vi "SingleStationGasMeter.vi"() -> ()   [LabVIEW 2014]
uses:
  <vilib>/DAQmx/read.llb/DAQmx Read (Analog 1D DBL NChan 1Samp).vi
panel:
  out "Meter 6 Present":bool
  out "Meter 5 Present":bool
  out "Meter 4 Present":bool
  out "Meter 3 Present":bool
  out "Meter 2 Present":bool
  out "Meter 1 Present":bool
  out "Meter Type 6":string
  out "Meter Type 2":string
  out "Meter Type 4":string
  out "Meter Type 5":string
  out "Meter Type 3":string
  out "Meter Type 1":string
  out "Meter 6 Size":dbl
  out "Meter 5 Size":dbl
  out "Meter 4 Size":dbl
  out "Meter 3 Size":dbl
  out "Meter 2 Size":dbl
  out "Meter 1 Size":dbl
  out "ANSI Placeholder":dbl
  out "Start Time ANSI":dbl
  in  "Start ANSI":bool
  out "ANSI 5 Minute Average (BTU/hr)":dbl format="%#_5g"
  out "30 Second Average (BTU/hr)":dbl format="%#_5g"
  out "15 Second Average (BTU/hr)":dbl format="%#_5g"
  out "Reference6":dbl
  out "Reference5":dbl
  out "Reference4":dbl
  out "Reference3":dbl
  out "Reference2":dbl
  out "Reference1":dbl
  out "Time":dbl
  out "Num Record":dbl
  in  "HeatingValueLP":dbl=2450.0 min=2400.0 max=2600.0 step=5.0
  out "Output 6":dbl min=0.0 max=5.0 step=0.01
  out "Output 5":dbl min=0.0 max=5.0 step=0.01
  out "Output 4":dbl min=0.0 max=5.0 step=0.01
  out "Output 3":dbl min=0.0 max=5.0 step=0.01
  out "Output 2":dbl min=0.0 max=5.0 step=0.01
  out "Output 1":dbl min=0.0 max=5.0 step=0.01
  out "Signal":bool
  in  "Record":bool
  out "File Path":path
  out "CF/HR":dbl format="%#_2g"
  out "HV":dbl
  in  "HeatingValueNG":dbl=990.0 min=990.0 max=1150.0 step=1.0
  out "Meter ID":dbl
  out "Gas":string
  out "DisplayChart":cluster{"Flow Rate":dbl}(graph)
  out "Flow Rate":dbl format="%#_5g"
  # "Instant Flow Rate (BTU/hr)"
  # "Heating Value"
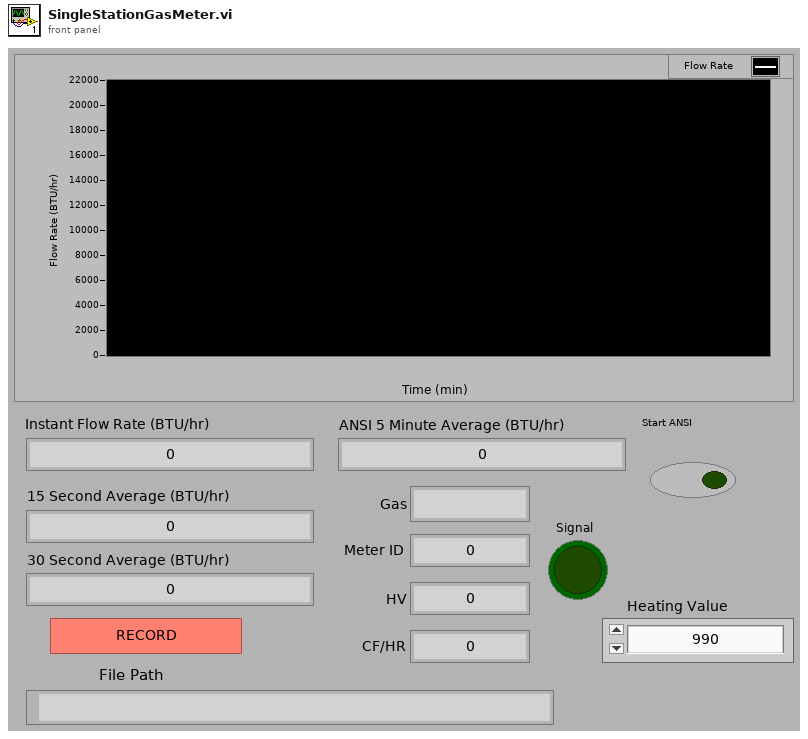
[diagram p1: front panel]
types:
  T1 = enum16{"open", "replace", "create", "open or create", "replace or create", "replace or create with confirmation"}
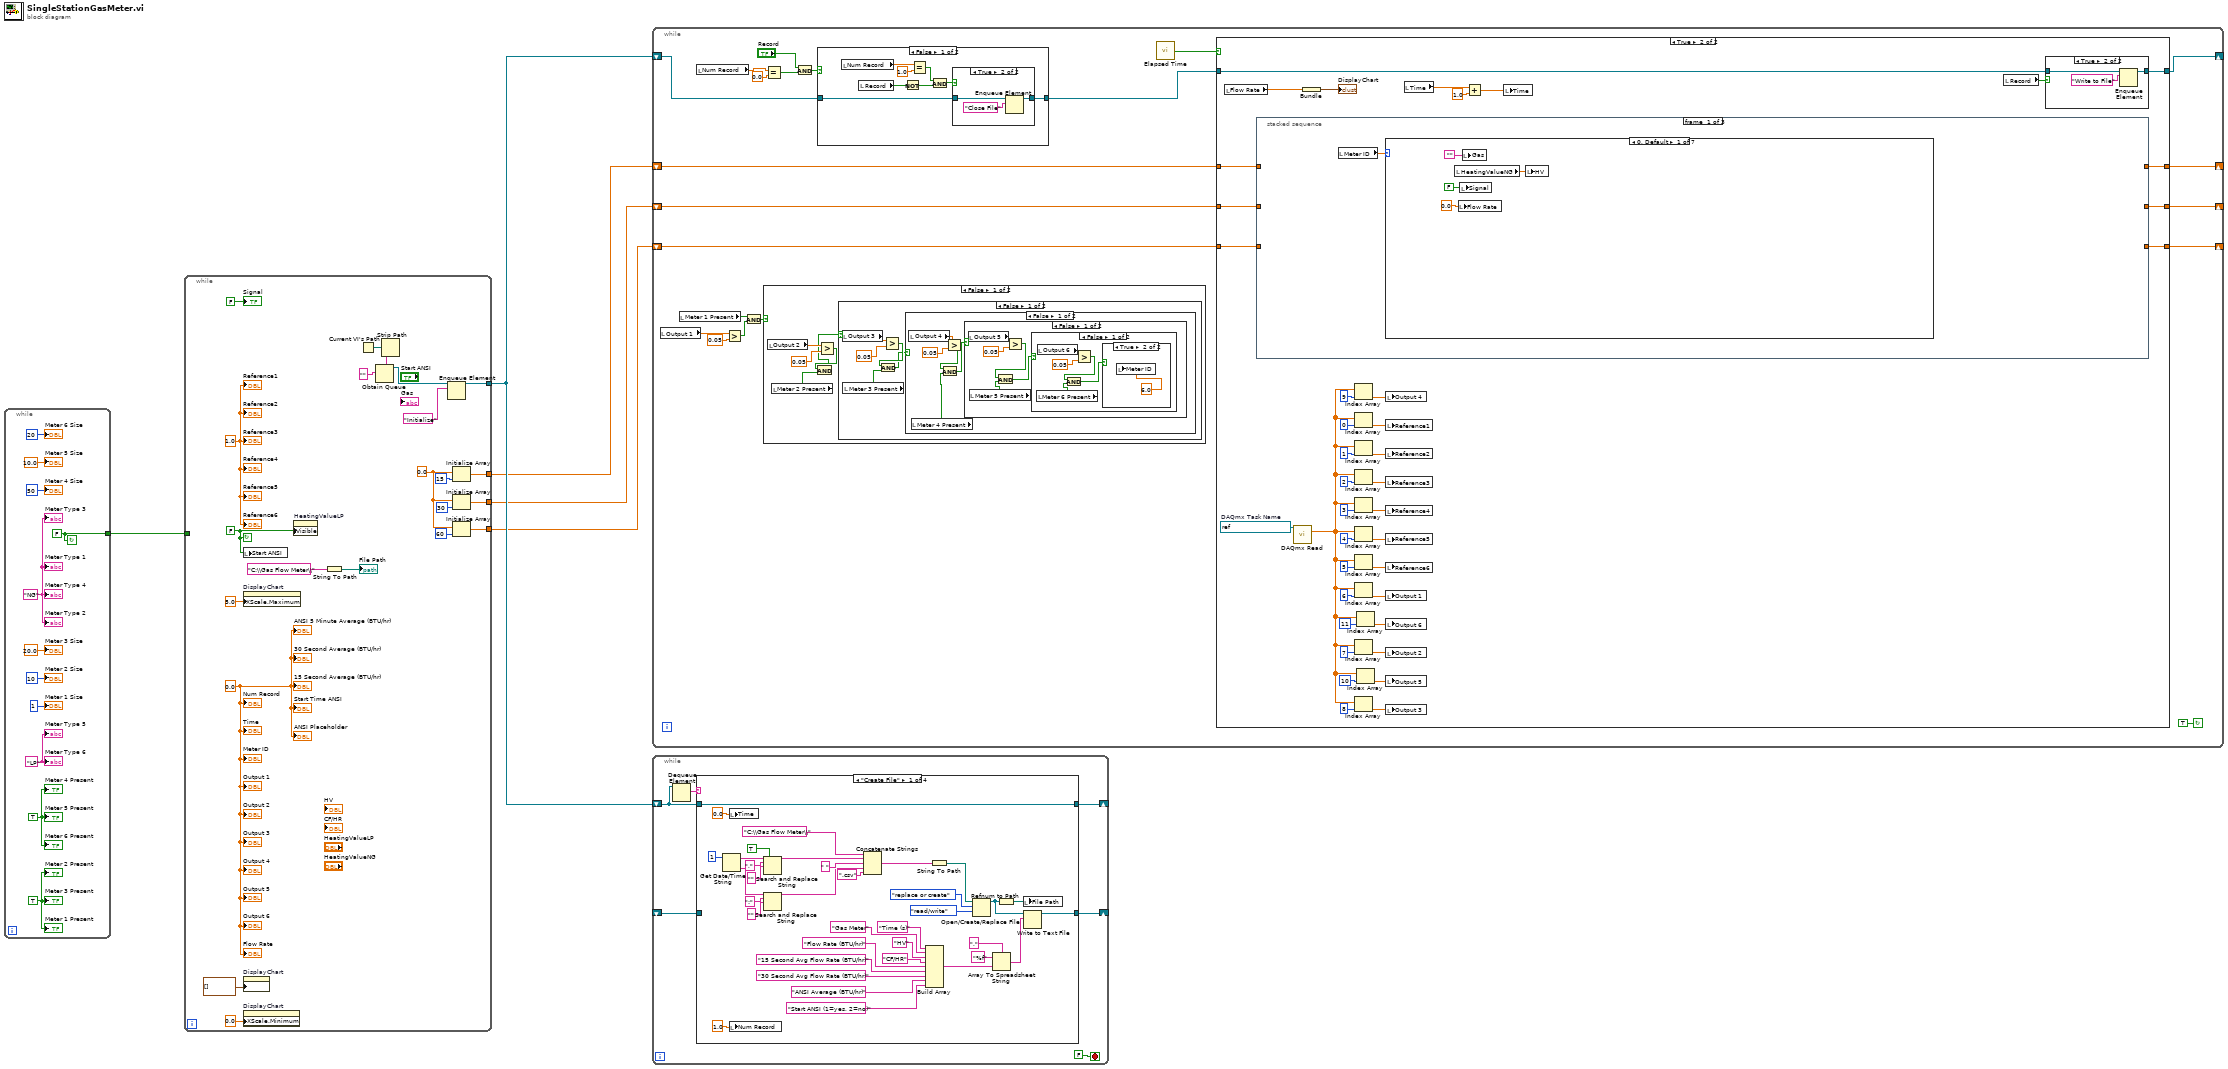
[diagram p0: block diagram]
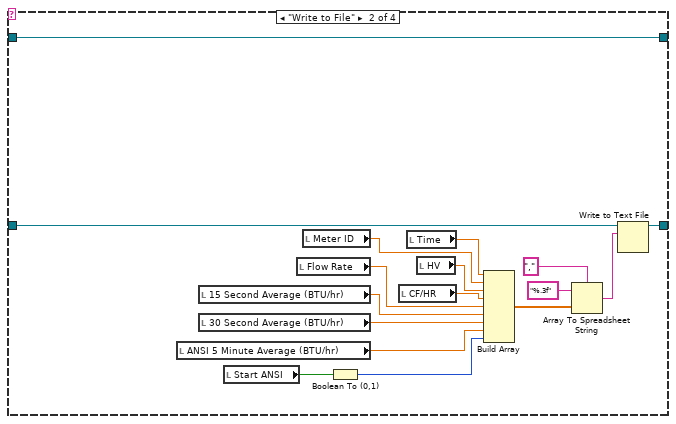
[diagram p2: hidden frame]
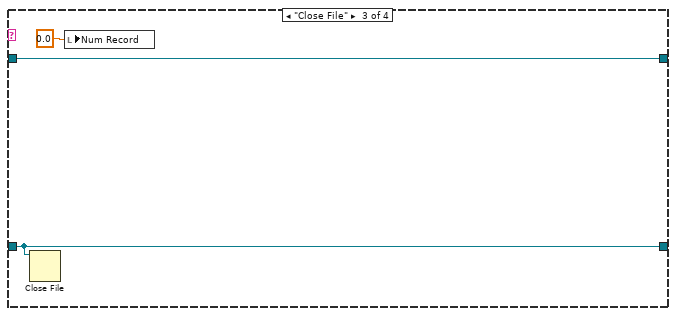
[diagram p3: hidden frame]
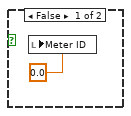
[diagram p5: hidden frame]
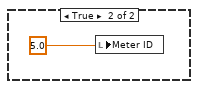
[diagram p6: hidden frame]
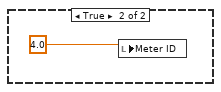
[diagram p7: hidden frame]
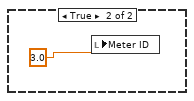
[diagram p8: hidden frame]
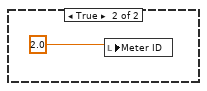
[diagram p9: hidden frame]
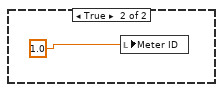
[diagram p10: hidden frame]
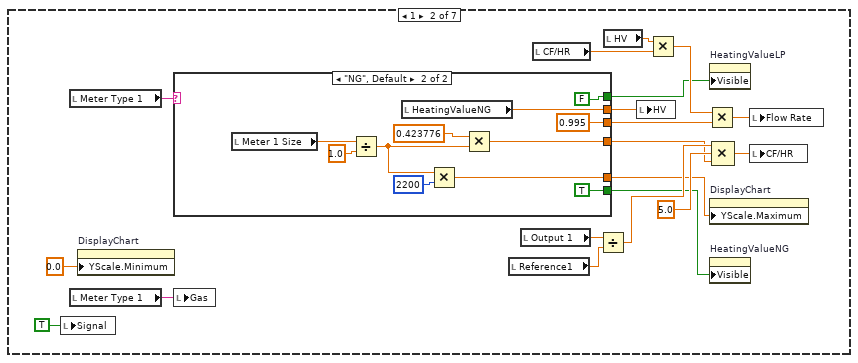
[diagram p12: hidden frame]
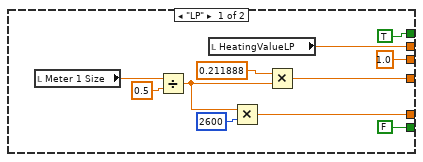
[diagram p13: hidden frame]
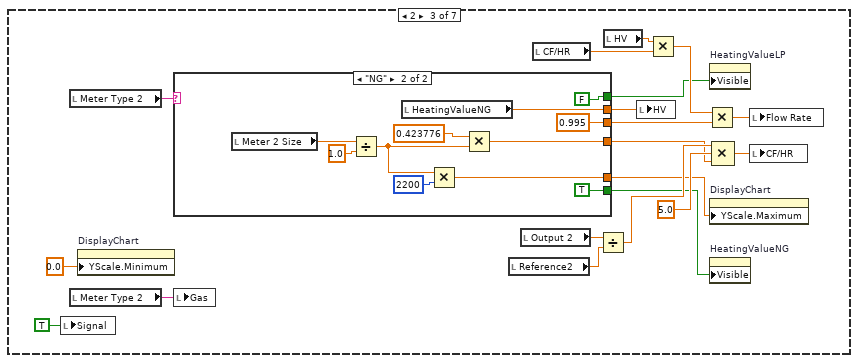
[diagram p14: hidden frame]
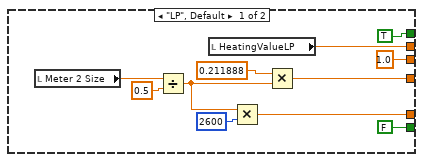
[diagram p15: hidden frame]
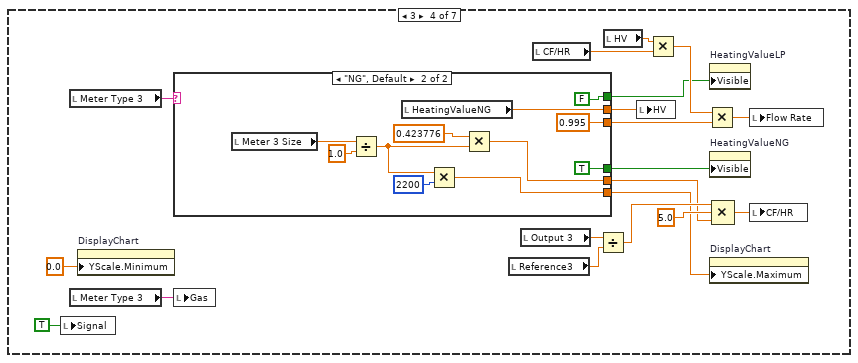
[diagram p16: hidden frame]
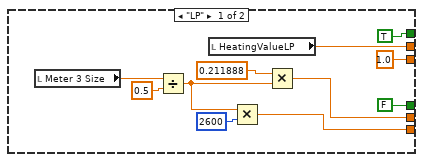
[diagram p17: hidden frame]
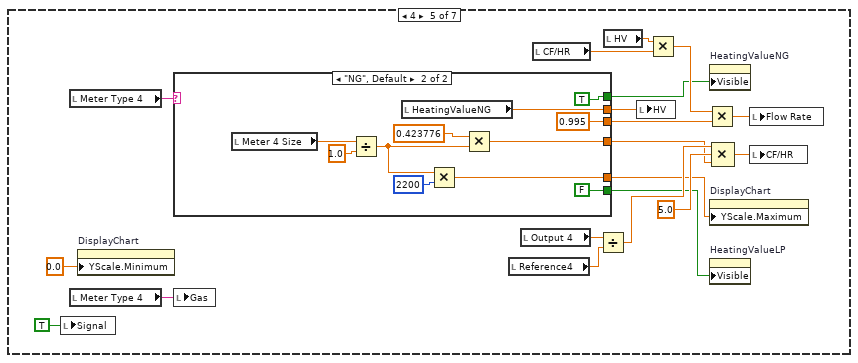
[diagram p18: hidden frame]
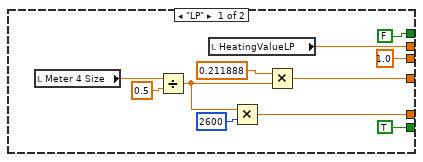
[diagram p19: hidden frame]
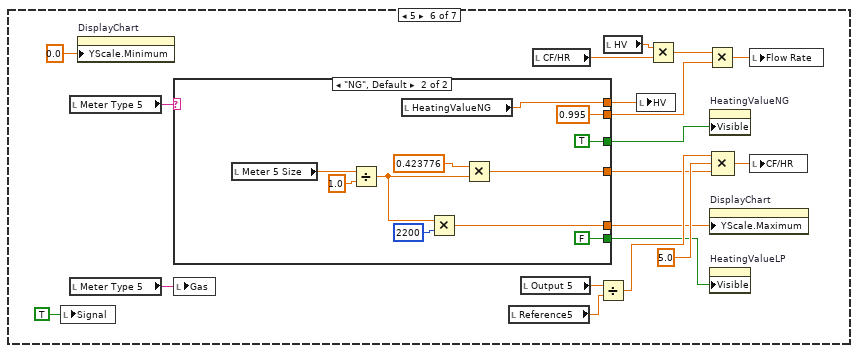
[diagram p20: hidden frame]
diagram:
  n1 = while {
    tunnel: [w16] -> w1
    stop <- w16 continue-if-true
    w13 = "LP"
    w6 = "NG"
    w14 = TRUE
    w15 = TRUE
    w16 = FALSE
    "Meter 4 Size" <- 50
    "Meter 5 Size" <- 10.0
    "Meter 2 Size" <- 10
    "Meter 1 Size" <- 1
    "Meter 6 Size" <- 20
    "Meter 3 Size" <- 20.0
    "Meter Type 1" <- w6
    "Meter Type 6" <- w13
    "Meter Type 3" <- w6
    "Meter Type 2" <- w6
    "Meter Type 5" <- w13
    "Meter Type 4" <- w6
    "Meter 1 Present" <- w15
    "Meter 2 Present" <- w15
    "Meter 3 Present" <- w15
    "Meter 4 Present" <- w14
    "Meter 5 Present" <- w14
    "Meter 6 Present" <- w14
  }
  n2 = while {
    tunnel: [w30] -> w5
    tunnel: [w24] -> w4
    tunnel: [w23] -> w3
    tunnel: [w20] -> w2
    tunnel: w1 -> [_]
    stop <- w19 continue-if-true
    w22 = 0.0
    w29 = 1.0
    w18 = 0.0
    w19 = FALSE
    n3 = local write "Start ANSI"(w19) -> ()
    n4 = property on="DisplayChart" class="WFChart (strict)"("XScale.Maximum"=5.0) -> ()  [unwired: 2 in, 2 out]
    n5 = property on="DisplayChart" class="WFChart (strict)"("History Data"=cluster{"[0]":dbl}[] []) -> ()  [unwired: 2 in, 2 out]
    n6 = property on="DisplayChart" class="WFChart (strict)"("XScale.Minimum"=0.0) -> ()  [unwired: 2 in, 2 out]
    n7 = property on="HeatingValueLP" class="DigNum (strict)"("Visible"=w19) -> ()  [unwired: 2 in, 2 out]
    n8 = String To Path(string="C:\\Gas Flow Meter\\") -> (path=→"File Path":path)
    n9 = Current VI's Path() -> (path=w35:path)
    n10 = Strip Path(path=w35) -> (name=w33:string)  [unwired: 1 out]
    n11 = Obtain Queue(name (unnamed)=w33, element data type="") -> (queue out=w31:refnum<queue>)  [unwired: 3 in, 2 out]
    n12 = Enqueue Element(queue=w31, element="Initialize") -> (queue out=w30:refnum<queue>)  [unwired: 2 in, 2 out]
    n13 = Initialize Array(w22, 15) -> (w24:dbl[])
    n14 = Initialize Array(w22, 30) -> (w23:dbl[])
    n15 = Initialize Array(w22, 60) -> (w20:dbl[])
    "Num Record" <- w18
    "Time" <- w18
    "Meter ID" <- w18
    "Output 1" <- w18
    "Output 2" <- w18
    "Output 3" <- w18
    "Output 4" <- w18
    "Output 5" <- w18
    "Output 6" <- w18
    "Reference1" <- w29
    "Reference2" <- w29
    "Reference3" <- w29
    "Reference4" <- w29
    "Reference5" <- w29
    "Reference6" <- w29
    "30 Second Average (BTU/hr)" <- w18
    "15 Second Average (BTU/hr)" <- w18
    "ANSI 5 Minute Average (BTU/hr)" <- w18
    "Start Time ANSI" <- w18
    "ANSI Placeholder" <- w18
    "Flow Rate" <- w18
    "Signal" <- FALSE
  }
  n16 = while {
    shift-right: [w51] -> _
    shift-left: w5 -> [w50]
    shift-right: [w47] -> _
    shift-left: w4 -> [w45]
    shift-right: [w46] -> _
    shift-left: w3 -> [w44]
    shift-right: [w43] -> _
    shift-left: w2 -> [w42]
    stop <- TRUE continue-if-true
    n17 = local read "Output 1"() -> (w49:dbl)
    n18 = local read "Meter 1 Present"() -> (w40:bool)
    n19 = local read "Num Record"() -> (w55:dbl)
    n20 = Greater?(x=w49, y=0.05) -> (0:w41:bool)
    n21 = And(x=w40, y=w41) -> (x .and. y?=w39:bool)
    n22 = case shown="False" w39 {
      frame False {
        n23 = local read "Output 2"() -> (w63:dbl)
        n24 = local read "Meter 2 Present"() -> (w62:bool)
        n25 = Greater?(x=w63, y=0.05) -> (0:w61:bool)
        n26 = And(x=w61, y=w62) -> (x .and. y?=w60:bool)
        n27 = case shown="False" w60 {
          frame False {
            n28 = local read "Output 3"() -> (w68:dbl)
            n29 = local read "Meter 3 Present"() -> (w67:bool)
            n30 = Greater?(x=w68, y=0.05) -> (0:w66:bool)
            n31 = And(x=w66, y=w67) -> (x .and. y?=w65:bool)
            n32 = case shown="False" w65 {
              frame False {
                n33 = local read "Output 4"() -> (w73:dbl)
                n34 = local read "Meter 4 Present"() -> (w72:bool)
                n35 = Greater?(x=w73, y=0.05) -> (0:w71:bool)
                n36 = And(x=w71, y=w72) -> (x .and. y?=w70:bool)
                n37 = case shown="False" w70 {
                  frame False {
                    n38 = local read "Output 5"() -> (w78:dbl)
                    n39 = local read "Meter 5 Present"() -> (w77:bool)
                    n40 = Greater?(x=w78, y=0.05) -> (0:w76:bool)
                    n41 = And(x=w76, y=w77) -> (x .and. y?=w75:bool)
                    n42 = case shown="False" w75 {
                      frame False {
                        n43 = local read "Meter 6 Present"() -> (w82:bool)
                        n44 = local read "Output 6"() -> (w83:dbl)
                        n45 = Greater?(x=w83, y=0.05) -> (0:w81:bool)
                        n46 = And(x=w81, y=w82) -> (x .and. y?=w80:bool)
                        n47 = case shown="True" w80 {
                          frame False {
                            n48 = local write "Meter ID"(0.0) -> ()
                          }
                          frame True {
                            n49 = local write "Meter ID"(6.0) -> ()
                          }
                        }
                      }
                      frame True {
                        n50 = local write "Meter ID"(5.0) -> ()
                      }
                    }
                  }
                  frame True {
                    n51 = local write "Meter ID"(4.0) -> ()
                  }
                }
              }
              frame True {
                n52 = local write "Meter ID"(3.0) -> ()
              }
            }
          }
          frame True {
            n53 = local write "Meter ID"(2.0) -> ()
          }
        }
      }
      frame True {
        n54 = local write "Meter ID"(1.0) -> ()
      }
    }
    n55 = Equal?(x=w55, y=0.0) -> (x = y?=w54:bool)
    n56 = And(x="Record", y=w54) -> (x .and. y?=w53:bool)
    n57 = case shown="False" w53 {
      tunnel: w50 -> [w435 w443]
      tunnel: [w434 w442] -> w52
      frame False {
        n58 = local read "Num Record"() -> (w437:dbl)
        n59 = local read "Record"() -> (w431:bool)
        n60 = Not(x=w431) -> (.not. x?=w430:bool)
        n61 = Equal?(x=w437, y=1.0) -> (x = y?=w433:bool)
        n62 = And(x=w433, y=w430) -> (x .and. y?=w432:bool)
        n63 = case shown="True" w432 {
          tunnel: w435 -> [w438 w440]
          tunnel: [w438 w439] -> w434
          frame False {
          }
          frame True {
            n64 = Enqueue Element(queue=w440, element="Close File") -> (queue out=w439:refnum<queue>)  [unwired: 2 in, 2 out]
          }
        }
      }
      frame True {
        n65 = Enqueue Element(queue=w443, element="Create File") -> (queue out=w442:refnum<queue>)  [unwired: 2 in, 2 out]
      }
    }
    n66 = call "Elapsed Time"() -> ("Time has Elapsed"=w58:bool)  [unwired: 12 in, 7 out]
    n67 = case shown="True" w58 {
      tunnel: w52 -> [w95 w129]
      tunnel: [w95 w128] -> w51
      tunnel: w45 -> [w94 w101]
      tunnel: w44 -> [w93 w100]
      tunnel: [w94 w99] -> w47
      tunnel: [w93 w98] -> w46
      tunnel: w42 -> [w92 w97]
      tunnel: [w92 w96] -> w43
      frame False {
      }
      frame True {
        w127 = refnum<k21> "ReadFlowMeterIn"  # DAQmx Task Name
        n68 = local read "Flow Rate"() -> (w135:dbl)
        n69 = stacked-sequence {
          tunnel: w101 -> [_ w411 _]
          tunnel: w100 -> [_ w410 _]
          tunnel: [_ w405 _] -> w99
          tunnel: [_ w401 _] -> w98
          tunnel: w97 -> [_ w395 _]
          tunnel: [_ w392 _] -> w96
          frame #0 {
            n70 = local read "Meter ID"() -> (w136:dbl)
            n71 = case shown="0, Default" w136 {
              frame 0, Default {
                n72 = local read "HeatingValueNG"() -> (w140:dbl)
                n73 = local write "Flow Rate"(0.0) -> ()
                n74 = local write "Signal"(FALSE) -> ()
                n75 = local write "Gas"("") -> ()
                n76 = local write "HV"(w140) -> ()
              }
              frame 1 {
                n77 = local write "Signal"(TRUE) -> ()
                n78 = local read "Meter Type 1"() -> (w149:string)
                n79 = local read "Meter Type 1"() -> (w143:string)
                n80 = property on="DisplayChart" class="WFChart (strict)"("YScale.Minimum"=0.0) -> ()  [unwired: 2 in, 2 out]
                n81 = case shown="\"NG\", Default" w149 {
                  tunnel: [w167 w178] -> w148
                  tunnel: [TRUE FALSE] -> w147
                  tunnel: [FALSE TRUE] -> w146
                  tunnel: [1.0 0.995] -> w145
                  tunnel: [w161 w172] -> w144
                  tunnel: [w160 w171] -> w142
                  frame "LP" {
                    n82 = local read "Meter 1 Size"() -> (w169:dbl)
                    n83 = Divide(x=w169, y=0.5) -> (x/y=w162:dbl)
                    n84 = local read "HeatingValueLP"() -> (w160:dbl)
                    n85 = Multiply(x=w162, y=2600) -> (x*y=w161:dbl)
                    n86 = Multiply(x=0.211888, y=w162) -> (x*y=w167:dbl)
                  }
                  frame "NG", Default {
                    n87 = local read "Meter 1 Size"() -> (w180:dbl)
                    n88 = Divide(x=w180, y=1.0) -> (x/y=w173:dbl)
                    n89 = local read "HeatingValueNG"() -> (w171:dbl)
                    n90 = Multiply(x=w173, y=2200) -> (x*y=w172:dbl)
                    n91 = Multiply(x=0.423776, y=w173) -> (x*y=w178:dbl)
                  }
                }
                n92 = local write "Gas"(w143) -> ()
                n93 = local read "Reference1"() -> (w153:dbl)
                n94 = local read "Output 1"() -> (w154:dbl)
                n95 = local read "CF/HR"() -> (w156:dbl)
                n96 = Divide(x=w154, y=w153) -> (x/y=w151:dbl)
                n97 = local read "HV"() -> (w155:dbl)
                n98 = local write "HV"(w142) -> ()
                n99 = Multiply(x=w155, y=w156) -> (x*y=w157:dbl)
                n100 = Multiply(x=w157, y=w145) -> (x*y=w158:dbl)
                n101 = property on="HeatingValueLP" class="DigNum (strict)"("Visible"=w147) -> ()  [unwired: 2 in, 2 out]
                n102 = property on="DisplayChart" class="WFChart (strict)"("YScale.Maximum"=w144) -> ()  [unwired: 2 in, 2 out]
                n103 = property on="HeatingValueNG" class="DigNum (strict)"("Visible"=w146) -> ()  [unwired: 2 in, 2 out]
                n104 = Compound Arithmetic op=MULTIPLY(w151, 5.0, w148) -> (w141:dbl)
                n105 = local write "Flow Rate"(w158) -> ()
                n106 = local write "CF/HR"(w141) -> ()
              }
              frame 2 {
                n107 = local write "Signal"(TRUE) -> ()
                n108 = local read "Meter Type 2"() -> (w190:string)
                n109 = local read "Meter Type 2"() -> (w184:string)
                n110 = property on="DisplayChart" class="WFChart (strict)"("YScale.Minimum"=0.0) -> ()  [unwired: 2 in, 2 out]
                n111 = case shown="\"NG\"" w190 {
                  tunnel: [w208 w219] -> w189
                  tunnel: [TRUE FALSE] -> w188
                  tunnel: [FALSE TRUE] -> w187
                  tunnel: [1.0 0.995] -> w186
                  tunnel: [w202 w213] -> w185
                  tunnel: [w201 w212] -> w183
                  frame "LP", Default {
                    n112 = local read "Meter 2 Size"() -> (w210:dbl)
                    n113 = Divide(x=w210, y=0.5) -> (x/y=w203:dbl)
                    n114 = local read "HeatingValueLP"() -> (w201:dbl)
                    n115 = Multiply(x=w203, y=2600) -> (x*y=w202:dbl)
                    n116 = Multiply(x=0.211888, y=w203) -> (x*y=w208:dbl)
                  }
                  frame "NG" {
                    n117 = local read "Meter 2 Size"() -> (w221:dbl)
                    n118 = Divide(x=w221, y=1.0) -> (x/y=w214:dbl)
                    n119 = local read "HeatingValueNG"() -> (w212:dbl)
                    n120 = Multiply(x=w214, y=2200) -> (x*y=w213:dbl)
                    n121 = Multiply(x=0.423776, y=w214) -> (x*y=w219:dbl)
                  }
                }
                n122 = local write "Gas"(w184) -> ()
                n123 = local read "Reference2"() -> (w194:dbl)
                n124 = local read "Output 2"() -> (w195:dbl)
                n125 = local read "CF/HR"() -> (w197:dbl)
                n126 = Divide(x=w195, y=w194) -> (x/y=w192:dbl)
                n127 = local read "HV"() -> (w196:dbl)
                n128 = local write "HV"(w183) -> ()
                n129 = Multiply(x=w196, y=w197) -> (x*y=w198:dbl)
                n130 = Multiply(x=w198, y=w186) -> (x*y=w199:dbl)
                n131 = property on="HeatingValueLP" class="DigNum (strict)"("Visible"=w188) -> ()  [unwired: 2 in, 2 out]
                n132 = property on="DisplayChart" class="WFChart (strict)"("YScale.Maximum"=w185) -> ()  [unwired: 2 in, 2 out]
                n133 = property on="HeatingValueNG" class="DigNum (strict)"("Visible"=w187) -> ()  [unwired: 2 in, 2 out]
                n134 = Compound Arithmetic op=MULTIPLY(w192, 5.0, w189) -> (w182:dbl)
                n135 = local write "Flow Rate"(w199) -> ()
                n136 = local write "CF/HR"(w182) -> ()
              }
              frame 3 {
                n137 = local write "Signal"(TRUE) -> ()
                n138 = local read "Meter Type 3"() -> (w231:string)
                n139 = local read "Meter Type 3"() -> (w225:string)
                n140 = property on="DisplayChart" class="WFChart (strict)"("YScale.Minimum"=0.0) -> ()  [unwired: 2 in, 2 out]
                n141 = case shown="\"NG\", Default" w231 {
                  tunnel: [w249 w260] -> w230
                  tunnel: [TRUE FALSE] -> w229
                  tunnel: [FALSE TRUE] -> w228
                  tunnel: [1.0 0.995] -> w227
                  tunnel: [w243 w254] -> w226
                  tunnel: [w242 w253] -> w224
                  frame "LP" {
                    n142 = local read "Meter 3 Size"() -> (w251:dbl)
                    n143 = Divide(x=w251, y=0.5) -> (x/y=w244:dbl)
                    n144 = local read "HeatingValueLP"() -> (w242:dbl)
                    n145 = Multiply(x=w244, y=2600) -> (x*y=w243:dbl)
                    n146 = Multiply(x=0.211888, y=w244) -> (x*y=w249:dbl)
                  }
                  frame "NG", Default {
                    n147 = local read "Meter 3 Size"() -> (w262:dbl)
                    n148 = Divide(x=w262, y=1.0) -> (x/y=w255:dbl)
                    n149 = local read "HeatingValueNG"() -> (w253:dbl)
                    n150 = Multiply(x=w255, y=2200) -> (x*y=w254:dbl)
                    n151 = Multiply(x=0.423776, y=w255) -> (x*y=w260:dbl)
                  }
                }
                n152 = local write "Gas"(w225) -> ()
                n153 = local read "Reference3"() -> (w235:dbl)
                n154 = local read "Output 3"() -> (w236:dbl)
                n155 = local read "CF/HR"() -> (w238:dbl)
                n156 = Divide(x=w236, y=w235) -> (x/y=w233:dbl)
                n157 = local read "HV"() -> (w237:dbl)
                n158 = local write "HV"(w224) -> ()
                n159 = Multiply(x=w237, y=w238) -> (x*y=w239:dbl)
                n160 = Multiply(x=w239, y=w227) -> (x*y=w240:dbl)
                n161 = property on="HeatingValueLP" class="DigNum (strict)"("Visible"=w229) -> ()  [unwired: 2 in, 2 out]
                n162 = property on="HeatingValueNG" class="DigNum (strict)"("Visible"=w228) -> ()  [unwired: 2 in, 2 out]
                n163 = property on="DisplayChart" class="WFChart (strict)"("YScale.Maximum"=w226) -> ()  [unwired: 2 in, 2 out]
                n164 = Compound Arithmetic op=MULTIPLY(w233, 5.0, w230) -> (w223:dbl)
                n165 = local write "Flow Rate"(w240) -> ()
                n166 = local write "CF/HR"(w223) -> ()
              }
              frame 4 {
                n167 = local write "Signal"(TRUE) -> ()
                n168 = local read "Meter Type 4"() -> (w272:string)
                n169 = local read "Meter Type 4"() -> (w266:string)
                n170 = property on="DisplayChart" class="WFChart (strict)"("YScale.Minimum"=0.0) -> ()  [unwired: 2 in, 2 out]
                n171 = case shown="\"NG\", Default" w272 {
                  tunnel: [w290 w301] -> w271
                  tunnel: [TRUE FALSE] -> w270
                  tunnel: [FALSE TRUE] -> w269
                  tunnel: [1.0 0.995] -> w268
                  tunnel: [w284 w295] -> w267
                  tunnel: [w283 w294] -> w265
                  frame "LP" {
                    n172 = local read "Meter 4 Size"() -> (w292:dbl)
                    n173 = Divide(x=w292, y=0.5) -> (x/y=w285:dbl)
                    n174 = local read "HeatingValueLP"() -> (w283:dbl)
                    n175 = Multiply(x=w285, y=2600) -> (x*y=w284:dbl)
                    n176 = Multiply(x=0.211888, y=w285) -> (x*y=w290:dbl)
                  }
                  frame "NG", Default {
                    n177 = local read "Meter 4 Size"() -> (w303:dbl)
                    n178 = Divide(x=w303, y=1.0) -> (x/y=w296:dbl)
                    n179 = local read "HeatingValueNG"() -> (w294:dbl)
                    n180 = Multiply(x=w296, y=2200) -> (x*y=w295:dbl)
                    n181 = Multiply(x=0.423776, y=w296) -> (x*y=w301:dbl)
                  }
                }
                n182 = local write "Gas"(w266) -> ()
                n183 = local read "Reference4"() -> (w276:dbl)
                n184 = local read "Output 4"() -> (w277:dbl)
                n185 = local read "CF/HR"() -> (w279:dbl)
                n186 = Divide(x=w277, y=w276) -> (x/y=w274:dbl)
                n187 = local read "HV"() -> (w278:dbl)
                n188 = local write "HV"(w265) -> ()
                n189 = Multiply(x=w278, y=w279) -> (x*y=w280:dbl)
                n190 = Multiply(x=w280, y=w268) -> (x*y=w281:dbl)
                n191 = property on="HeatingValueNG" class="DigNum (strict)"("Visible"=w269) -> ()  [unwired: 2 in, 2 out]
                n192 = property on="DisplayChart" class="WFChart (strict)"("YScale.Maximum"=w267) -> ()  [unwired: 2 in, 2 out]
                n193 = property on="HeatingValueLP" class="DigNum (strict)"("Visible"=w270) -> ()  [unwired: 2 in, 2 out]
                n194 = Compound Arithmetic op=MULTIPLY(w274, 5.0, w271) -> (w264:dbl)
                n195 = local write "Flow Rate"(w281) -> ()
                n196 = local write "CF/HR"(w264) -> ()
              }
              frame 5 {
                n197 = local write "Signal"(TRUE) -> ()
                n198 = local read "Meter Type 5"() -> (w313:string)
                n199 = local read "Meter Type 5"() -> (w307:string)
                n200 = property on="DisplayChart" class="WFChart (strict)"("YScale.Minimum"=0.0) -> ()  [unwired: 2 in, 2 out]
                n201 = case shown="\"NG\", Default" w313 {
                  tunnel: [w331 w342] -> w312
                  tunnel: [TRUE FALSE] -> w311
                  tunnel: [FALSE TRUE] -> w310
                  tunnel: [1.0 0.995] -> w309
                  tunnel: [w325 w336] -> w308
                  tunnel: [w324 w335] -> w306
                  frame "LP" {
                    n202 = local read "Meter 5 Size"() -> (w333:dbl)
                    n203 = Divide(x=w333, y=0.5) -> (x/y=w326:dbl)
                    n204 = local read "HeatingValueLP"() -> (w324:dbl)
                    n205 = Multiply(x=w326, y=2600) -> (x*y=w325:dbl)
                    n206 = Multiply(x=0.211888, y=w326) -> (x*y=w331:dbl)
                  }
                  frame "NG", Default {
                    n207 = local read "Meter 5 Size"() -> (w344:dbl)
                    n208 = Divide(x=w344, y=1.0) -> (x/y=w337:dbl)
                    n209 = local read "HeatingValueNG"() -> (w335:dbl)
                    n210 = Multiply(x=w337, y=2200) -> (x*y=w336:dbl)
                    n211 = Multiply(x=0.423776, y=w337) -> (x*y=w342:dbl)
                  }
                }
                n212 = local write "Gas"(w307) -> ()
                n213 = local read "Reference5"() -> (w317:dbl)
                n214 = local read "Output 5"() -> (w318:dbl)
                n215 = local read "CF/HR"() -> (w320:dbl)
                n216 = Divide(x=w318, y=w317) -> (x/y=w315:dbl)
                n217 = local read "HV"() -> (w319:dbl)
                n218 = local write "HV"(w306) -> ()
                n219 = Multiply(x=w319, y=w320) -> (x*y=w321:dbl)
                n220 = Multiply(x=w321, y=w309) -> (x*y=w322:dbl)
                n221 = property on="HeatingValueNG" class="DigNum (strict)"("Visible"=w310) -> ()  [unwired: 2 in, 2 out]
                n222 = property on="DisplayChart" class="WFChart (strict)"("YScale.Maximum"=w308) -> ()  [unwired: 2 in, 2 out]
                n223 = property on="HeatingValueLP" class="DigNum (strict)"("Visible"=w311) -> ()  [unwired: 2 in, 2 out]
                n224 = Compound Arithmetic op=MULTIPLY(w315, 5.0, w312) -> (w305:dbl)
                n225 = local write "Flow Rate"(w322) -> ()
                n226 = local write "CF/HR"(w305) -> ()
              }
              frame 6 {
                n227 = local write "Signal"(TRUE) -> ()
                n228 = local read "Meter Type 6"() -> (w354:string)
                n229 = local read "Meter Type 6"() -> (w348:string)
                n230 = property on="DisplayChart" class="WFChart (strict)"("YScale.Minimum"=0.0) -> ()  [unwired: 2 in, 2 out]
                n231 = case shown="\"NG\", Default" w354 {
                  tunnel: [w372 w383] -> w353
                  tunnel: [TRUE FALSE] -> w352
                  tunnel: [FALSE TRUE] -> w351
                  tunnel: [1.0 0.995] -> w350
                  tunnel: [w366 w377] -> w349
                  tunnel: [w365 w376] -> w347
                  frame "LP" {
                    n232 = local read "Meter 6 Size"() -> (w374:dbl)
                    n233 = Divide(x=w374, y=0.5) -> (x/y=w367:dbl)
                    n234 = local read "HeatingValueLP"() -> (w365:dbl)
                    n235 = Multiply(x=w367, y=2600) -> (x*y=w366:dbl)
                    n236 = Multiply(x=0.211888, y=w367) -> (x*y=w372:dbl)
                  }
                  frame "NG", Default {
                    n237 = local read "Meter 6 Size"() -> (w385:dbl)
                    n238 = Divide(x=w385, y=1.0) -> (x/y=w378:dbl)
                    n239 = local read "HeatingValueNG"() -> (w376:dbl)
                    n240 = Multiply(x=w378, y=2200) -> (x*y=w377:dbl)
                    n241 = Multiply(x=0.423776, y=w378) -> (x*y=w383:dbl)
                  }
                }
                n242 = local write "Gas"(w348) -> ()
                n243 = local read "Reference6"() -> (w358:dbl)
                n244 = local read "Output 6"() -> (w359:dbl)
                n245 = local read "CF/HR"() -> (w361:dbl)
                n246 = Divide(x=w359, y=w358) -> (x/y=w356:dbl)
                n247 = local read "HV"() -> (w360:dbl)
                n248 = local write "HV"(w347) -> ()
                n249 = Multiply(x=w360, y=w361) -> (x*y=w362:dbl)
                n250 = Multiply(x=w362, y=w350) -> (x*y=w363:dbl)
                n251 = property on="HeatingValueNG" class="DigNum (strict)"("Visible"=w351) -> ()  [unwired: 2 in, 2 out]
                n252 = property on="DisplayChart" class="WFChart (strict)"("YScale.Maximum"=w349) -> ()  [unwired: 2 in, 2 out]
                n253 = property on="HeatingValueLP" class="DigNum (strict)"("Visible"=w352) -> ()  [unwired: 2 in, 2 out]
                n254 = Compound Arithmetic op=MULTIPLY(w356, 5.0, w353) -> (w346:dbl)
                n255 = local write "Flow Rate"(w363) -> ()
                n256 = local write "CF/HR"(w346) -> ()
              }
            }
          }
          frame #1 {
            n257 = Delete From Array(array=w411, index=14) -> (array with subset deleted=w406:dbl[])  [unwired: 1 in, 1 out]
            n258 = Delete From Array(array=w410, index=29) -> (array with subset deleted=w407:dbl[])  [unwired: 1 in, 1 out]
            n259 = Delete From Array(array=w395, index=59) -> (array with subset deleted=w393:dbl[])  [unwired: 1 in, 1 out]
            n260 = local read "Flow Rate"() -> (w388:dbl)
            n261 = Insert Into Array(array=w406, index=0, new element=w388) -> (w405:dbl[])
            n262 = Insert Into Array(array=w407, index=0, new element=w388) -> (w401:dbl[])
            n263 = Insert Into Array(array=w393, index=0, new element=w388) -> (w392:dbl[])
            n264 = Add Array Elements(numeric array=w405) -> (sum=w403:dbl)
            n265 = Add Array Elements(numeric array=w401) -> (sum=w400:dbl)
            n266 = Add Array Elements(numeric array=w392) -> (sum=w391:dbl)
            n267 = Array Size(array=w405) -> (size(s)=w404:i32)
            n268 = Array Size(array=w401) -> (size(s)=w399:i32)
            n269 = Array Size(array=w392) -> (size(s)=w390:i32)
            n270 = Divide(x=w403, y=w404) -> (x/y=w402:dbl)
            n271 = Divide(x=w400, y=w399) -> (x/y=w398:dbl)
            n272 = Divide(x=w391, y=w390) -> (x/y=w389:dbl)
            n273 = local write "15 Second Average (BTU/hr)"(w402) -> ()
            n274 = local write "30 Second Average (BTU/hr)"(w398) -> ()
            n275 = local write "ANSI Placeholder"(w389) -> ()
          }
          frame #2 {
            n276 = local read "Start ANSI"() -> (w412:bool)
            n277 = case shown="True" w412 {
              frame False {
              }
              frame True {
                n278 = local read "Start Time ANSI"() -> (w414:dbl)
                n279 = Equal?(x=w414, y=0.0) -> (x = y?=w413:bool)
                n280 = case shown="False" w413 {
                  frame False {
                    n281 = local read "Start Time ANSI"() -> (w420:dbl)
                    n282 = Add(x=w420, y=360) -> (x+y=w418:dbl)
                    n283 = local read "Time"() -> (w417:dbl)
                    n284 = Less Or Equal?(x=w417, y=w418) -> (x <= y?=w416:bool)
                    n285 = case shown="False" w416 {
                      frame False {
                        n286 = local write "Start Time ANSI"(0.0) -> ()
                        n287 = local write "Start ANSI"(FALSE) -> ()
                        n288 = local read "ANSI Placeholder"() -> (w422:dbl)
                        n289 = local write "ANSI 5 Minute Average (BTU/hr)"(w422) -> ()
                      }
                      frame True {
                      }
                    }
                  }
                  frame True {
                    n290 = local read "Time"() -> (w425:dbl)
                    n291 = local write "ANSI 5 Minute Average (BTU/hr)"(0.0) -> ()
                    n292 = local write "Start Time ANSI"(w425) -> ()
                  }
                }
              }
            }
          }
        }
        n293 = call-poly <vilib>:"DAQmx Read.vi"("task/channels in"=w127) -> ("data"=w126:dbl[])  [unwired: 12 in, 2 out]
        n294 = Bundle("Flow Rate"=w135) -> (→"DisplayChart":cluster{"Flow Rate":dbl})  [unwired: 1 in]
        n295 = Index Array(array=w126, index=9) -> (element=w111:dbl)
        n296 = Index Array(array=w126, index=0) -> (element=w102:dbl)
        n297 = Index Array(array=w126, index=1) -> (element=w103:dbl)
        n298 = Index Array(array=w126, index=2) -> (element=w104:dbl)
        n299 = Index Array(array=w126, index=3) -> (element=w105:dbl)
        n300 = Index Array(array=w126, index=4) -> (element=w106:dbl)
        n301 = Index Array(array=w126, index=5) -> (element=w107:dbl)
        n302 = Index Array(array=w126, index=6) -> (element=w108:dbl)
        n303 = Index Array(array=w126, index=7) -> (element=w109:dbl)
        n304 = Index Array(array=w126, index=8) -> (element=w110:dbl)
        n305 = Index Array(array=w126, index=11) -> (element=w113:dbl)
        n306 = Index Array(array=w126, index=10) -> (element=w112:dbl)
        n307 = local write "Output 4"(w111) -> ()
        n308 = local write "Reference1"(w102) -> ()
        n309 = local write "Reference2"(w103) -> ()
        n310 = local write "Reference3"(w104) -> ()
        n311 = local write "Reference4"(w105) -> ()
        n312 = local write "Reference5"(w106) -> ()
        n313 = local write "Reference6"(w107) -> ()
        n314 = local write "Output 1"(w108) -> ()
        n315 = local write "Output 6"(w113) -> ()
        n316 = local write "Output 2"(w109) -> ()
        n317 = local write "Output 5"(w112) -> ()
        n318 = local write "Output 3"(w110) -> ()
        n319 = local read "Time"() -> (w131:dbl)
        n320 = Add(x=w131, y=1.0) -> (x+y=w130:dbl)
        n321 = local write "Time"(w130) -> ()
        n322 = local read "Record"() -> (w133:bool)
        n323 = case shown="True" w133 {
          tunnel: w129 -> [w426 w428]
          tunnel: [w426 w427] -> w128
          frame False {
          }
          frame True {
            n324 = Enqueue Element(queue=w428, element="Write to File") -> (queue out=w427:refnum<queue>)  [unwired: 2 in, 2 out]
          }
        }
      }
    }
  }
  n325 = while {
    shift-right: [w448] -> _
    shift-left: w5 -> [w445]
    shift-right: [w447] -> _
    shift-left: _ -> [w446]
    stop <- FALSE stop-if-true
    n326 = Dequeue Element(queue=w445) -> (element=w449:string)  [unwired: 2 in, 3 out]
    n327 = case shown="\"Create File\"" w449 {
      tunnel: [w456 w494 w505 w508] -> w448
      tunnel: w445 -> [w456 w494 w505 w508]
      tunnel: [w455 w492 w504 w507] -> w447
      tunnel: w446 -> [_ w493 w504 w507]
      frame "Create File" {
        n328 = Get Date/Time String(date format (0)=1) -> (date string=w461:string, time string=w458:string)  [unwired: 2 in]
        n329 = local write "Time"(0.0) -> ()
        n330 = local write "Num Record"(1.0) -> ()
        n331 = Search and Replace String(input string=w458, search string=":", replace string="") -> (result string=w467:string)  [unwired: 5 in, 3 out]
        n332 = Search and Replace String(replace all?=TRUE, input string=w461, search string=",", replace string="") -> (result string=w468:string)  [unwired: 4 in, 3 out]
        n333 = Concatenate Strings("C:\\Gas Flow Meter\\", w468, " ", w467, ".csv") -> (w464:string)
        n334 = Build Array("Time (s)", "Gas Meter", "HV", "CF/HR", "Flow Rate (BTU/hr)", "15 Second Avg Flow Rate (BTU/hr)", "30 Second Avg Flow Rate (BTU/hr)", "ANSI Average (BTU/hr)", "Start ANSI (1=yes, 2=no)") -> (w478:string[])
        n335 = String To Path(string=w464) -> (path=w484:path)
        n336 = Open/Create/Replace File(file path (use dialog)=w484, operation (0:open)=T1."replace or create", access (0:read/write)=enum16{"read/write", "read-only", "write-only"}."read/write") -> (refnum out=w486:refnum<file>)  [unwired: 3 in, 2 out]
        n337 = Array To Spreadsheet String(delimiter (Tab)=",", array=w478, 3:"%f" ("format string")) -> (spreadsheet string=w479:string)
        n338 = Refnum to Path(1:w486) -> (0:w485:path)
        n339 = local write "File Path"(w485) -> ()
        n340 = Write to Text File(file (use dialog)=w486, text=w479) -> (refnum out=w455:refnum<file>)  [unwired: 2 in, 2 out]
      }
      frame "Write to File" {
        n341 = local read "ANSI 5 Minute Average (BTU/hr)"() -> (w489:dbl)
        n342 = local read "15 Second Average (BTU/hr)"() -> (w490:dbl)
        n343 = local read "30 Second Average (BTU/hr)"() -> (w491:dbl)
        n344 = local read "Start ANSI"() -> (w488:bool)
        n345 = local read "Flow Rate"() -> (w497:dbl)
        n346 = local read "Meter ID"() -> (w500:dbl)
        n347 = Boolean To (0,1)(Boolean=w488) -> (0, 1=w487:i16)
        n348 = local read "CF/HR"() -> (w498:dbl)
        n349 = local read "Time"() -> (w501:dbl)
        n350 = local read "HV"() -> (w499:dbl)
        n351 = Build Array(w501, w500, w499, w498, w497, w490, w491, w489, w487) -> (w496:dbl[])
        n352 = Array To Spreadsheet String(delimiter (Tab)=",", array=w496, 3:"%.3f" ("format string")) -> (spreadsheet string=w495:string)
        n353 = Write to Text File(file (use dialog)=w493, text=w495) -> (refnum out=w492:refnum<file>)  [unwired: 2 in, 2 out]
      }
      frame "Close File" {
        n354 = Close File(refnum=w504) -> ()  [unwired: 1 in, 2 out]
        n355 = local write "Num Record"(0.0) -> ()
      }
      frame "Initialize", Default {
      }
    }
  }
